vi "myRIO_BRig_RT_dataCurrent_IfirstTrial.vi"() -> (2 "output_I_firstTrial":i32)   [LabVIEW 2014]
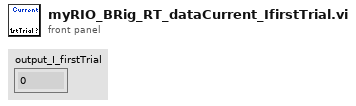
[diagram p1: front panel]
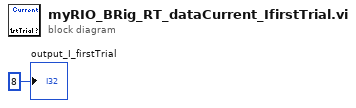
[diagram p0: block diagram]
diagram:
  "output_I_firstTrial" <- 8 ("output_iBlock")
